vi "左右转.vi"(1 "目标角度":dbl, 2 "当前角度":dbl) -> (0 "左转/右转":bool)   [LabVIEW 2016]
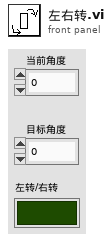
[diagram p1: front panel]
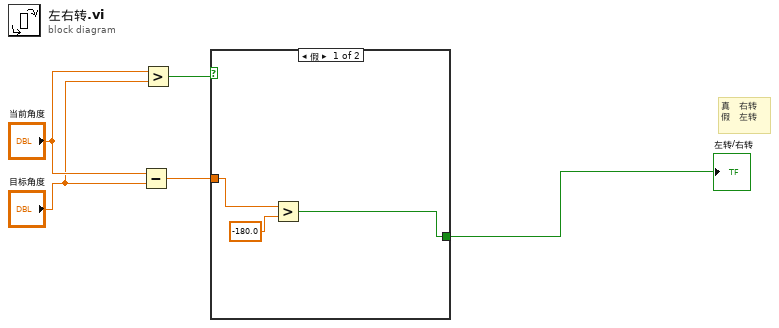
[diagram p0: block diagram]
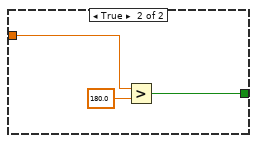
[diagram p2: hidden frame]
diagram:
  # "真   右转\n假   左转"
  n1 = Subtract(x="当前角度", y="目标角度") -> (x-y=w2:dbl)
  n2 = Greater?(x="当前角度", y="目标角度") -> (0:w3:bool)
  n3 = case shown="假" w3 {
    tunnel: w2 -> [w8 w10]
    tunnel: [w6 w9] -> w1
    frame False {
      n4 = Greater?(x=w8, y=-180.0) -> (0:w6:bool)
    }
    frame True {
      n5 = Greater?(x=w10, y=180.0) -> (0:w9:bool)
    }
  }
  "左转/右转" <- w1
